vi "Fetch Multi Eval Meas List ES Flatness Ripple Results.vi"(7 "Result Type (Current)":i32(ring) items=["Current", "Average", "Extreme", "Standard Deviation"], 8 "error in (no error)":errorcluster, 9 "Ripple (Ripple 1)":T1=1 items=["Ripple 1"=1, "Ripple 2"=2], 10 "Instance (1)":T2=1, 11 "VISA resource name":refnum<visa-resource-name>) -> (0 "error out":errorcluster, 1 "ES Flatness Ripple Results":dbl[](array[numeric]) format="%^.3e", 2 "Reliability":i32, 3 "VISA resource name out":refnum<visa-resource-name>)   [LabVIEW 2015, in "Rohde&Schwarz CMXP NR FR2 Measurement.lvlib"]
doc: "Returns equalizer spectrum flatness single value results (ripple 1 or ripple 2) for all measured list mode segments.\n\nAttributes:\nRSCMXPNRFR2M_ATTR_FETCH_MULTI_EVAL_MEASUREMENT_LIST_ESF_RIPPLE_AVERAGE_RESULTS\nRSCMXPNRFR2M_ATTR_FETCH_MULTI_EVAL_MEASUREMENT_LIST_ESF_RIPPLE_CURRENT_RESULTS\nRSCMXPNRFR2M_ATTR_FETCH_MULTI_EVAL_MEASUREMENT_LIST_ESF_RIPPLE_EXTREME_RESULTS\nRSCMXPNRFR2M_ATTR_FETCH_MULTI_EVAL_MEASUREMENT_LIST_ESF_RIPPLE_STANDARD_DEVIATION_RESULTS\n\nRemote-control commands:\nFETCh:NRMMw:MEAS<i>:MEValuation:LIST:ESFLatness:RIPPle<no>:AVERage?\nFETCh:NRMMw:MEAS<i>:MEValuation:LIST:ESFLatness:RIPPle<no>:CURRent?\nFETCh:NRMMw:MEAS<i>:MEValuation:LIST:ESFLatness:RIPPle<no>:EXTReme?\nFETCh:NRMMw:MEAS<i>:MEValuation:LIST:ESFLatness:RIPPle<no>:SDEViation?"
uses:
  <instrlib>/Rohde&Schwarz CMXP NR FR2 Measurement/Rohde&Schwarz CMXP NR FR2 Measurement.lvlib
  <instrlib>/Rohde&Schwarz CMXP NR FR2 Measurement/Private/_Instance.ctl
  <instrlib>/Rohde&Schwarz CMXP NR FR2 Measurement/Private/_Ripple.ctl
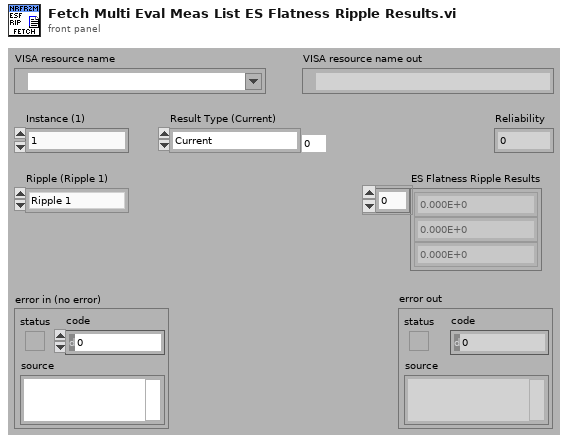
[diagram p1: front panel]
types:
  T1 = typedef "Rohde&Schwarz CMXP NR FR2 Measurement.lvlib/_Ripple.ctl" = i32
  T2 = typedef "Rohde&Schwarz CMXP NR FR2 Measurement.lvlib/_Instance.ctl" = i32
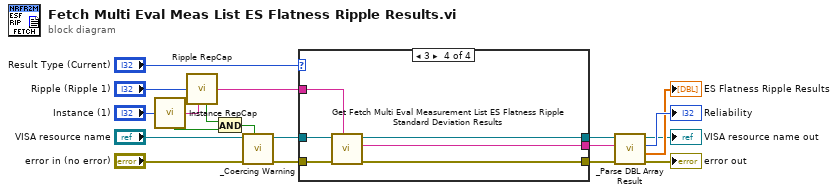
[diagram p0: block diagram]
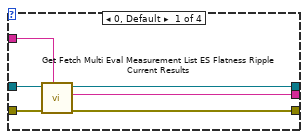
[diagram p2: hidden frame]
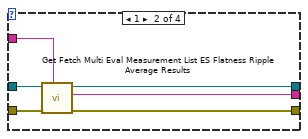
[diagram p3: hidden frame]
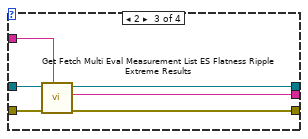
[diagram p4: hidden frame]
diagram:
  n1 = call <instrlib>:"Instance RepCap.vi"("Instance In"="Instance (1)") -> ("In Range?"=w17:bool, "RepCap Identifier Out"=w1:string)  [unwired: 1 in]
  n2 = call <instrlib>:"Ripple RepCap.vi"("Ripple In"="Ripple (Ripple 1)", "RepCap String In (\"\")"=w1) -> ("In Range?"=w19:bool, "RepCap Identifier Out"=w10:string)
  n3 = And(x=w19, y=w17) -> (x .and. y?=w18:bool)
  n4 = call <instrlib>:"_Coercing Warning.vi"("In Range?"=w18, "error in (no error)"="error in (no error)", "VISA resource name"="VISA resource name") -> ("error out"=w12:errorcluster, "VISA resource name out"=w11:refnum<visa-resource-name>)  [unwired: 7 in]
  n5 = case shown="3" "Result Type (Current)" {
    tunnel: w12 -> [w25 w31 w37 w43]
    tunnel: w11 -> [w24 w30 w36 w42]
    tunnel: w10 -> [w23 w29 w35 w41]
    tunnel: [w22 w28 w34 w40] -> w8
    tunnel: [w21 w27 w33 w39] -> w7
    tunnel: [w20 w26 w32 w38] -> w6
    frame 0, Default {
      n6 = call "Get Fetch Multi Eval Measurement List ES Flatness Ripple Current Results"("Repeated Capabilities"=w23, "error in (no error)"=w25, "instrument handle"=w24) -> ("error out"=w22:errorcluster, "Fetch Multi Eval Measurement List ES Flatness Ripple Current Results"=w21:string, "instrument handle out"=w20:refnum<visa-resource-name>)  [unwired: 6 in]
    }
    frame 1 {
      n7 = call "Get Fetch Multi Eval Measurement List ES Flatness Ripple Average Results"("Repeated Capabilities"=w29, "error in (no error)"=w31, "instrument handle"=w30) -> ("error out"=w28:errorcluster, "Fetch Multi Eval Measurement List ES Flatness Ripple Average Results"=w27:string, "instrument handle out"=w26:refnum<visa-resource-name>)  [unwired: 6 in]
    }
    frame 2 {
      n8 = call "Get Fetch Multi Eval Measurement List ES Flatness Ripple Extreme Results"("Repeated Capabilities"=w35, "error in (no error)"=w37, "instrument handle"=w36) -> ("error out"=w34:errorcluster, "Fetch Multi Eval Measurement List ES Flatness Ripple Extreme Results"=w33:string, "instrument handle out"=w32:refnum<visa-resource-name>)  [unwired: 6 in]
    }
    frame 3 {
      n9 = call "Get Fetch Multi Eval Measurement List ES Flatness Ripple Standard Deviation Results"("Repeated Capabilities"=w41, "error in (no error)"=w43, "instrument handle"=w42) -> ("error out"=w40:errorcluster, "Fetch Multi Eval Measurement List ES Flatness Ripple Standard Deviation Results"=w39:string, "instrument handle out"=w38:refnum<visa-resource-name>)  [unwired: 6 in]
    }
  }
  n10 = call <instrlib>:"_Parse DBL Array Result.vi"("error in (no error)"=w8, "Input String"=w7, "VISA resource name"=w6) -> ("error out"=→"error out":errorcluster, "Results"=→"ES Flatness Ripple Results":dbl[], "Reliability"=→"Reliability":i32, "VISA resource name out"=→"VISA resource name out":refnum<visa-resource-name>)  [unwired: 5 in]
